vi "dfd_Params (N,a,b) to k.vi"(0 "order":i32, 2 "passband ripple":dbl format="%.2f", 3 "stopband attenuation":dbl format="%.2f") -> (4 "e":dbl format="%.4f", 5 "Elliptic Primes":cluster{"snc":dbl, "cnc":dbl, "dnc":dbl} {"dnc" format="%.2f"; "cnc" format="%.2f"; "snc" format="%.2f"}, 6 "k":dbl format="%.4f", 7 "K":dbl format="%.4f", 8 "k'":dbl format="%.4f", 9 "K'":dbl format="%.4f")   [LabVIEW 2017, in "NI_DigFilter_Design.lvlib"]
uses:
  <vilib>/addons/Digital Filter Design/NI_DigFilter_Design.lvlib
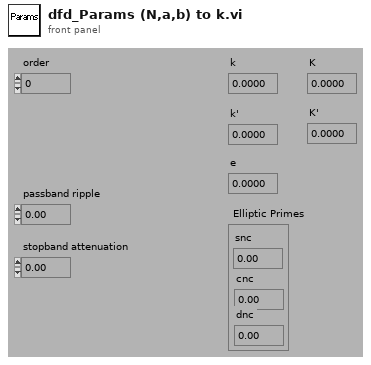
[diagram p1: front panel]
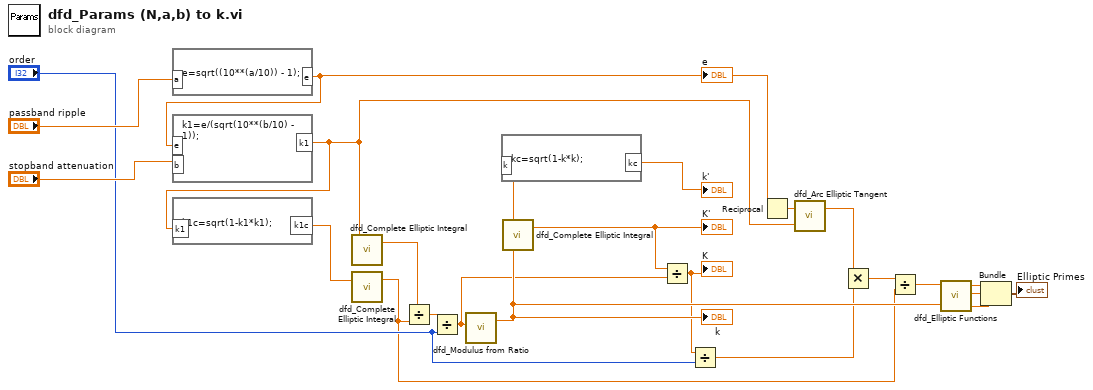
[diagram p0: block diagram]
diagram:
  n1 = formula code="e=sqrt((10**(a/10)) - 1);"("a"="passband ripple") -> ("e"=w13:dbl)
  "e" <- w13
  n2 = formula code="k1=e/(sqrt(10**(b/10) - 1));"("e"=w13, "b"="stopband attenuation") -> ("k1"=w11:dbl)
  n3 = formula code="k1c=sqrt(1-k1*k1);"("k1"=w11) -> ("k1c"=w21:dbl)
  n4 = call <vilib>:"dfd_Complete Elliptic Integral.vi"("k'"=w11) -> ("cei(k)"=w20:dbl)  [unwired: 1 out]
  n5 = call <vilib>:"dfd_Complete Elliptic Integral.vi"("k'"=w21) -> ("cei(k)"=w8:dbl)  [unwired: 1 out]
  n6 = Divide(x=w20, y=w8) -> (x/y=w19:dbl)
  n7 = Divide(x=w19, y="order") -> (x/y=w16:dbl)
  n8 = call <vilib>:"dfd_Modulus from Ratio.vi"("u"=w16) -> ("fk(u)"=w18:dbl)  [unwired: 1 out]
  "k" <- w18
  n9 = formula code="kc=sqrt(1-k*k);"("k"=w18) -> ("kc"=→"k'":dbl)
  n10 = call <vilib>:"dfd_Complete Elliptic Integral.vi"("k'"=w18) -> ("cei(k)"=w17:dbl)  [unwired: 1 out]
  "K'" <- w17
  n11 = Divide(x=w17, y=w16) -> (x/y=w15:dbl)
  "K" <- w15
  n12 = Divide(x=w15, y="order") -> (x/y=w10:dbl)
  n13 = Reciprocal(x=w13) -> (1/x=w12:dbl)
  n14 = call <vilib>:"dfd_Arc Elliptic Tangent.vi"("k'"=w11, "u"=w12) -> ("arcsc(u,k)"=w9:dbl)  [unwired: 1 out]
  n15 = Multiply(x=w9, y=w10) -> (x*y=w7:dbl)
  n16 = Divide(x=w7, y=w8) -> (x/y=w6:dbl)
  n17 = call <vilib>:"dfd_Elliptic Functions.vi"("u"=w6, "k'"=w18) -> ("sn(k)"=w5:dbl, "cn(k)"=w4:dbl, "dn(k)"=w3:dbl)  [unwired: 1 out]
  n18 = Bundle("sn(k)"=w5, "cn(k)"=w4, "dn(k)"=w3) -> (→"Elliptic Primes":cluster{"sn(k)":dbl, "cn(k)":dbl, "dn(k)":dbl})  [unwired: 1 out]
